vi "Subscribe to Results.vi"(8 "error in (no error)":errorcluster, 10 "Result Observer":refnum<class "Result Observer.lvclass">, 11 "Single Thread Test Runner In":refnum<class "Single Thread Test Runner.lvclass">) -> (0 "error out":errorcluster, 3 "Single Thread Test Runner Out":refnum<class "Single Thread Test Runner.lvclass">)   [LabVIEW 2020, in "Single Thread Test Runner.lvclass"]
uses:
  Single Thread Test Runner.lvclass
  Result Observer/Result Observer.lvclass
  Single Thread Test Runner.lvclass/Single Thread Test Runner.ctl
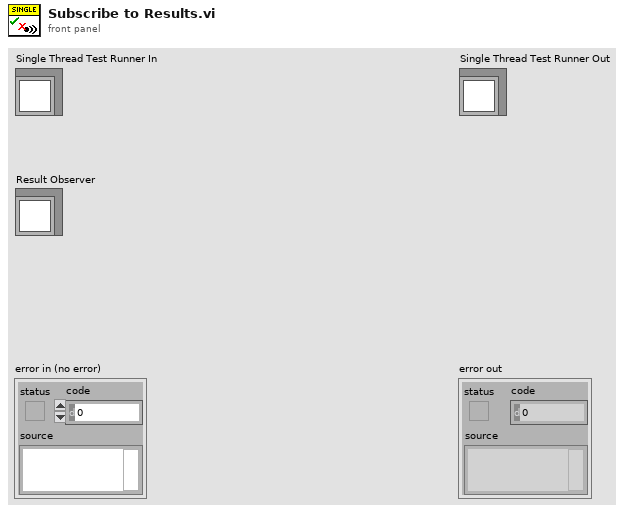
[diagram p1: front panel]
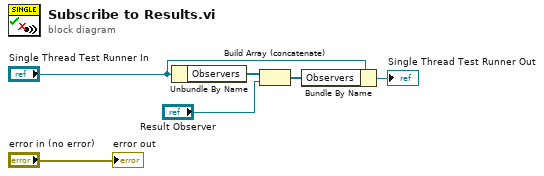
[diagram p0: block diagram]
diagram:
  n1 = Unbundle By Name("Single Thread Test Runner In") -> ("Observers"=w4:refnum<class "Result Observer.lvclass">[])
  n2 = Build Array (concatenate)(w4, "Result Observer") -> (w1:refnum<class "Result Observer.lvclass">[])
  n3 = Bundle By Name(cluster="Single Thread Test Runner In", "Observers"=w1) -> (→"Single Thread Test Runner Out":refnum<class "Single Thread Test Runner.lvclass">)
  "error out" <- "error in (no error)"
